vi "Measurement Logic.vi"() -> ()   [LabVIEW 2021, in "Noise Sweep_Class D Amplifier.lvlib"]
uses:
  Noise Sweep_Class D Amplifier.lvlib
  Measurement Configuration.ctl
  shared/DAQmx/input terminal configuration.ctl
  shared/controls/weighting filter.ctl
  Measurement Results.ctl
  <vilib>/MeasurementLink/MeasurementLink Measurement Server/Measure Call Context/Measure Call Context.lvclass
  <instrlib>/niDCPower/nidcpower.llb/niDCPower Source Mode.ctl
  <instrlib>/niDCPower/nidcpower.llb/niDCPower Output Function.ctl
  <instrlib>/niDCPower/nidcpower.llb/niDCPower Wait For Event - Event.ctl
  <vilib>/Analysis/1siggen.llb/Ramp Pattern by Samples.vi
  <vilib>/Analysis/5stat.llb/RMS (DBL).vi
  <vilib>/DAQmx/create/channels.llb/DAQmx Create Channel (AI-Voltage-Basic).vi
  <vilib>/DAQmx/configure/timing.llb/DAQmx Timing (Sample Clock).vi
  <vilib>/addons/Sound and Vibration/svt_Weighting/SVT A, B, C Weighting Filter (Fixed Rates) (N Ch).vi
  <vilib>/Analysis/NI_AALBase.lvlib
  <vilib>/addons/Sound and Vibration/svt_Weighting/SoundVib_ABCWeighting.lvlib
  <vilib>/Analysis/NI_AALPro.lvlib
  shared/DAQmx/DAQmx utility.lvlib
panel:
  out "XY Graph":cluster{"X data":dbl[], "Y data":dbl[]}[](graph)
  out "Waveform Graph":waveform(dbl)[](graph)
  out "measure call context out":refnum<class "Measure Call Context.lvclass">
  in  "measure call context in":refnum<class "Measure Call Context.lvclass">
  out "measurement results":T1={"channel names"=[], "power supply voltage (V)"=[], "idle channel noise (Vrms)"=[], "wfm - dt"=1.9531249997269942e-05, "wfm - data"=array[12800 elements]}
  in  "measurement configuration":T2={"acq channel"="PXI1Slot4/ai0", "acq sampling rate"=51200.0, "measurement time (s)"=0.1, "input range"=5.0, "input terminal cfg"=enum."Default", "weighting filter"=enum."A-weighting", "power supply resource"="PXI1Slot6", "power supply voltage start"=5.0, "power supply voltage stop"=14.0, "sweep number of steps"=10, "power supply current limit"=1.2}
  out "error out":errorcluster
  in  "error in":errorcluster
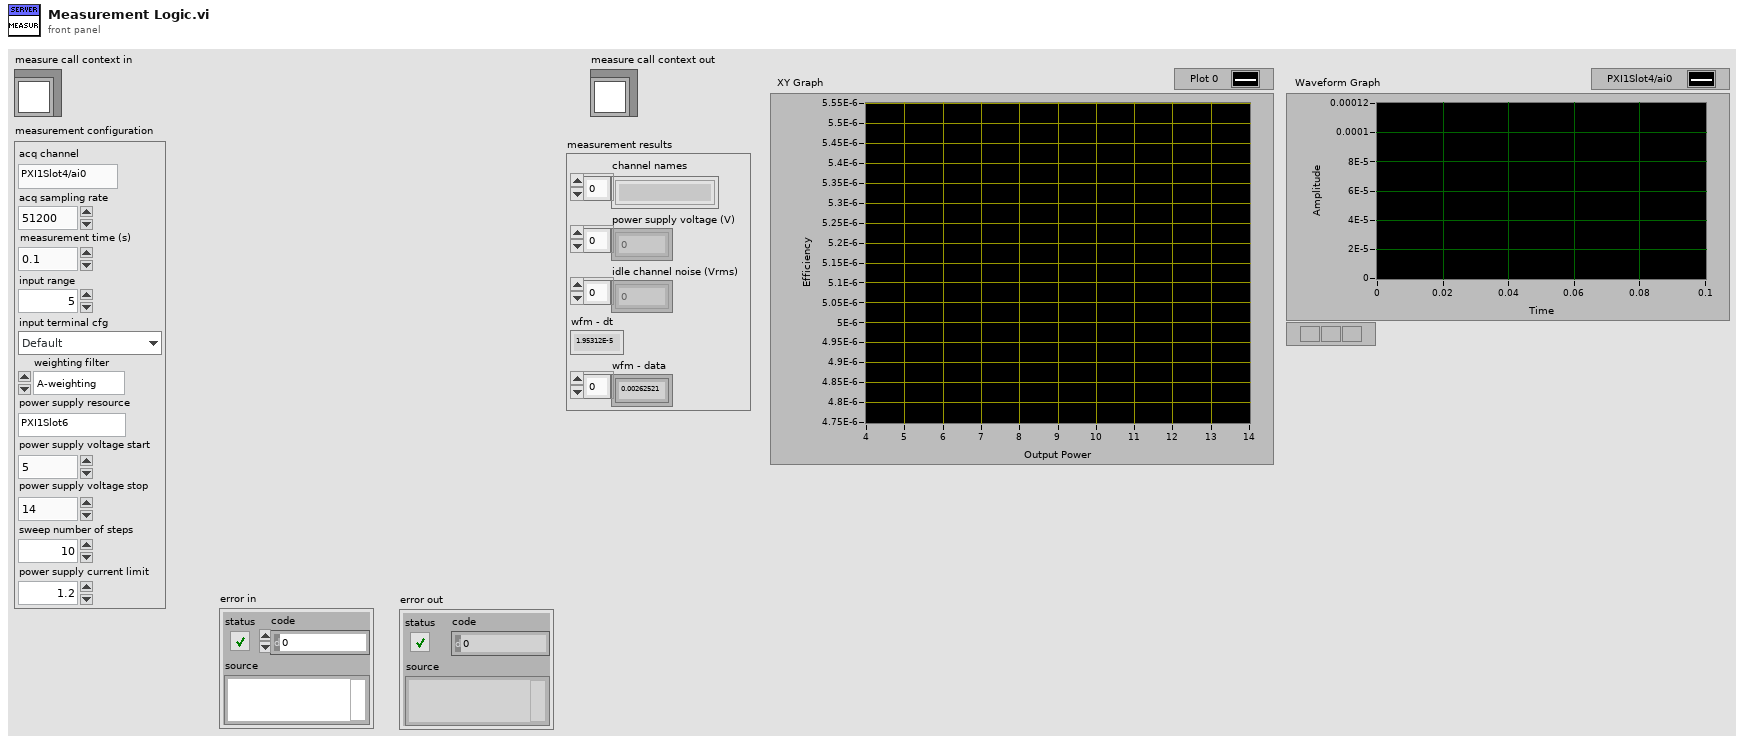
[diagram p1: front panel]
types:
  T1 = typedef "Noise Sweep_Class D Amplifier.lvlib/Measurement Results.ctl" = cluster{"channel names":string[], "power supply voltage (V)":dbl[], "idle channel noise (Vrms)":dbl[], "wfm - dt":dbl, "wfm - data":dbl[]}
  T2 = typedef "Noise Sweep_Class D Amplifier.lvlib/Measurement Configuration.ctl" = cluster{"acq channel":string, "acq sampling rate":dbl, "measurement time (s)":dbl, "input range":dbl, "input terminal cfg":T3, "weighting filter":T4, "power supply resource":string, "power supply voltage start":dbl, "power supply voltage stop":dbl, "sweep number of steps":u32, "power supply current limit":dbl}
  T3 = typedef "DAQmx utility.lvlib/input terminal configuration.ctl" = enum32{"Default", "NRSE", "RSE", "Differential", "Pseudodifferential"}
  T4 = typedef "weighting filter.ctl" = enum32{"Linear", "A-weighting", "B-weighting", "C-weighting"}
  T5 = typedef "niDCPower Output Function.ctl" = i32
  T6 = typedef "niDCPower Source Mode.ctl" = i32
  T7 = typedef "niDCPower Wait For Event - Event.ctl" = i32
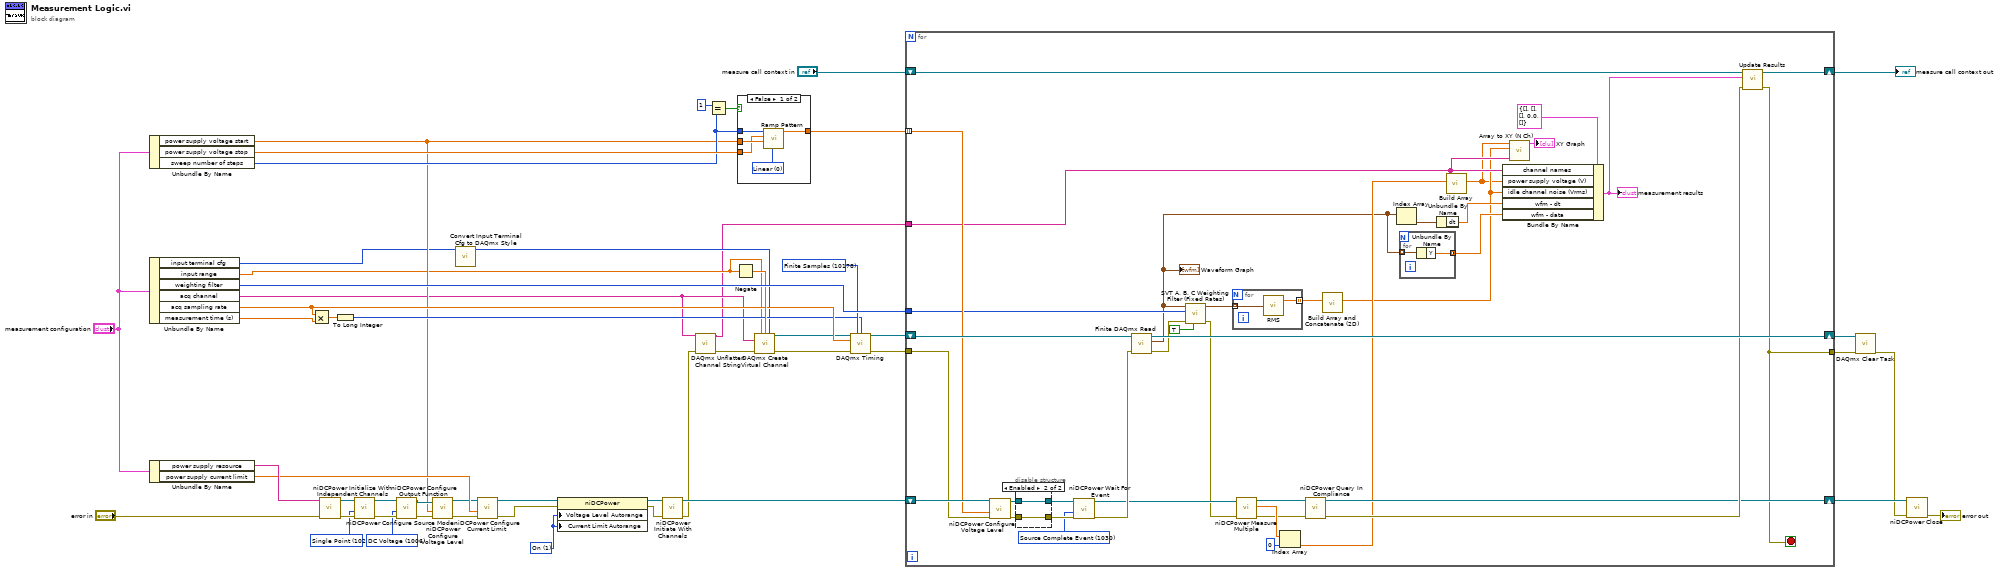
[diagram p0: block diagram]
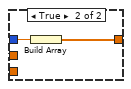
[diagram p2: hidden frame]
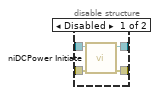
[diagram p3: hidden frame]
diagram:
  w18 = 10178 items=["Finite Samples"=10178, "Continuous Samples"=10123, "Hardware Timed Single Point"=12522] ("sample mode")
  w24 = 1 items=["Off", "On"] ("Source:DC Voltage:Current Limit Autorange")
  w25 = T5 1006 items=["DC Voltage"=1006, "DC Current"=1007, "Pulse Voltage"=1049, "Pulse Current"=1050] ("output function")
  w32 = T6 1020 items=["Single Point"=1020, "Sequence"=1021] ("source mode")
  n1 = Unbundle By Name("measurement configuration") -> ("power supply voltage start"=w12:dbl, "power supply voltage stop"=w23:dbl, "sweep number of steps"=w22:u32)
  n2 = Unbundle By Name("measurement configuration") -> ("input terminal cfg"=w9:T3, "input range"=w11:dbl, "weighting filter"=w21:T4, "acq channel"=w2:string, "acq sampling rate"=w16:dbl, "measurement time (s)"=w17:dbl)
  n3 = Unbundle By Name("measurement configuration") -> ("power supply resource"=w46:string, "power supply current limit"=w45:dbl)
  n4 = Multiply(x=w16, y=w17) -> (x*y=w15:dbl)
  n5 = call <instrlib>:"niDCPower Initialize With Independent Channels.vi"("error in (no error)"="error in", "resource name"=w46) -> ("error out"=w36:errorcluster, "instrument handle out"=w35:refnum<k15>)  [unwired: 8 in]
  n6 = To Long Integer(number=w15) -> (32bit integer=w14:i32)
  n7 = call <instrlib>:"niDCPower Configure Source Mode.vi"("error in (no error)"=w36, "source mode"=w32, "instrument handle"=w35) -> ("error out"=w34:errorcluster, "instrument handle out"=w33:refnum<k15>)  [unwired: 7 out]
  n8 = call <instrlib>:"niDCPower Configure Output Function.vi"("error in (no error)"=w34, "output function"=w25, "instrument handle"=w33) -> ("error out"=w26:errorcluster, "instrument handle out"=w27:refnum<k15>)  [unwired: 1 in, 6 out]
  n9 = call <instrlib>:"niDCPower Configure Voltage Level.vi"("error in (no error)"=w26, "voltage level"=w12, "instrument handle"=w27) -> ("error out"=w37:errorcluster, "instrument handle out"=w38:refnum<k15>)  [unwired: 1 in, 6 out]
  n10 = call "Convert Input Terminal Cfg to DAQmx Style.vi"("input terminal cfg"=w9) -> ("DAQmx input terminal cfg"=w10:i32)  [unwired: 10 in]
  n11 = call <instrlib>:"niDCPower Configure Current Limit.vi"("error in (no error)"=w37, "current limit"=w45, "instrument handle"=w38) -> ("error out"=w28:errorcluster, "instrument handle out"=w31:refnum<k15>)  [unwired: 2 in, 5 out]
  n12 = property class="niDCPower"(reference=w31, error in=w28, "Voltage Level Autorange"=w24, "Current Limit Autorange"=w24) -> (reference out=w30:refnum<k15>, error out=w29:errorcluster)
  n13 = call <instrlib>:"niDCPower Initiate With Channels.vi"("error in (no error)"=w29, "instrument handle"=w30) -> ("error out"=w4:errorcluster, "instrument handle out"=w41:refnum<k15>)  [unwired: 8 in]
  n14 = call <vilib>:"DAQmx Unflatten Channel String.vi"("names in"=w2, "error in"=w4) -> ("names out"=w1:string[], "error out"=w3:errorcluster)  [unwired: 12 in]
  n15 = Equal?(x=u32 1, y=w22) -> (x = y?=w49:bool)
  n16 = Negate(x=w11) -> (-x=w19:dbl)
  n17 = case shown="False" w49 {
    tunnel: w12 -> [w56 w58]
    tunnel: w23 -> [w55 _]
    tunnel: w22 -> [w54 _]
    tunnel: [w53 w57] -> w51
    frame False {
      w52 = u16 0 items=["Linear", "Logarithmic"] ("type")
      n18 = call-poly <vilib>:"Ramp Pattern.vi"("type"=w52, "start"=w56, "end"=w55, "samples"=w54) -> ("Ramp Pattern"=w53:dbl[])  [unwired: 6 in, 1 out]
    }
    frame True {
      n19 = Build Array(w58) -> (w57:dbl[])
    }
  }
  n20 = call-poly <vilib>:"DAQmx Create Virtual Channel.vi"("maximum value"=w11, "minimum value"=w19, "input terminal configuration"=w10, "physical channels"=w2, "error in"=w3) -> ("task out"=w8:refnum<k21>, "error out"=w7:errorcluster)  [unwired: 9 in]
  n21 = call-poly <vilib>:"DAQmx Timing.vi"("task/channels in"=w8, "sample mode"=w18, "samples per channel"=w14, "rate"=w16, "error in"=w7) -> ("task out"=w6:refnum<k21>, "error out"=w5:errorcluster)  [unwired: 9 in]
  n22 = for {
    tunnel: w51 -> [w86] mode=indexing
    shift-right: [w96] -> w50
    shift-left: "measure call context in" -> [w95]
    shift-right: [w75] -> w42
    shift-left: w41 -> [w88]
    shift-right: [w93] -> w40
    shift-left: w6 -> [w92]
    tunnel: w5 -> [w87]
    tunnel: w21 -> [w72]
    tunnel: [w71] -> w13
    tunnel: w1 -> [w62]
    stop <- w71 stop-if-true
    w83 = T7 1030 items=["Source Complete Event"=1030, "Measure Complete Event"=1031, "Sequence Iteration Complete Event"=1032, "Sequence Engine Done Event"=1033] ("event")
    n23 = call <instrlib>:"niDCPower Configure Voltage Level.vi"("error in (no error)"=w87, "voltage level"=w86, "instrument handle"=w88) -> ("error out"=w82:errorcluster, "instrument handle out"=w81:refnum<k15>)  [unwired: 1 in, 6 out]
    n24 = disable-structure shown="Enabled" {
      disable-tunnel: [w102 w104] -> w85
      disable-tunnel: [w101 w103] -> w84
      disable-tunnel: w82 -> [w100 w103]
      disable-tunnel: w81 -> [w99 w104]
      frame Disabled {
        n25 = call <instrlib>:"niDCPower Initiate.vi"("error in (no error)"=w100, "instrument handle"=w99) -> ("error out"=w101:errorcluster, "instrument handle out"=w102:refnum<k15>)  [unwired: 2 in, 6 out]
      }
      frame Enabled {
      }
    }
    n26 = call <instrlib>:"niDCPower Wait For Event.vi"("error in (no error)"=w84, "event"=w83, "instrument handle"=w85) -> ("error out"=w80:errorcluster, "instrument handle out"=w79:refnum<k15>)  [unwired: 1 in, 6 out]
    n27 = call "Finite DAQmx Read.vi"("error in (no error)"=w80, "task/channels in"=w92) -> ("error out"=w74:errorcluster, "data"=w65:waveform(dbl)[], "task out"=w93:refnum<k21>)  [unwired: 7 in]
    "Waveform Graph" <- w65
    n28 = call-poly <vilib>:"SVT A, B, C Weighting Filter (Fixed Rates).vi"("reset filter (F)"=TRUE, "error in (no error)"=w74, "weighting"=w72, "scaled signals [EU]"=w65) -> ("error out"=w73:errorcluster, "weighted signals [EU]"=w69:waveform(dbl)[])  [unwired: 5 in]
    n29 = for {
      tunnel: w69 -> [w106] mode=indexing
      tunnel: [w105] -> w63 mode=indexing
      n30 = call-poly <vilib>:"RMS.vi"("X"=w106) -> ("rms value"=w105:dbl)  [unwired: 1 out]
    }
    n31 = call <instrlib>:"niDCPower Measure Multiple.vi"("error in (no error)"=w73, "instrument handle"=w79) -> ("error out"=w78:errorcluster, "voltage measurements"=w89:dbl[], "instrument handle out"=w76:refnum<k15>)  [unwired: 6 in, 1 out]
    n32 = Index Array(array=w89, index=0) -> (element=w67:dbl)
    n33 = call <instrlib>:"niDCPower Query In Compliance.vi"("error in (no error)"=w78, "instrument handle"=w76) -> ("error out"=w77:errorcluster, "instrument handle out"=w75:refnum<k15>)  [unwired: 1 in, 7 out]
    n34 = call "Build Array and Concatenate (2D).vi"("Array"=w63) -> ("Array Out"=w60:dbl[])  [unwired: 10 in]
    n35 = Index Array(array=w65) -> (element=w68:waveform(dbl))  [unwired: 1 in]
    n36 = for {
      tunnel: w65 -> [w98] mode=indexing
      tunnel: [w97] -> w64 mode=concatenating
      n37 = Unbundle By Name(w98) -> ("Y"=w97:dbl[])
    }
    n38 = Unbundle By Name(w68) -> ("dt"=w66:dbl)
    n39 = call "Build Array.vi"("value"=w67) -> ("Array"=w59:dbl[])  [unwired: 10 in]
    n40 = Bundle By Name(cluster=T1 {"channel names"=[], "power supply voltage (V)"=[], "idle channel noise (Vrms)"=[], "wfm - dt"=0.0, "wfm - data"=[]} ("Measurement Results"), "channel names"=w62, "power supply voltage (V)"=w59, "idle channel noise (Vrms)"=w60, "wfm - dt"=w66, "wfm - data"=w64) -> (w94:T1)
    "measurement results" <- w94
    n41 = call "Array to XY (N Ch).vi"("channel names"=w62, "Y data"=w60, "X data"=w59) -> ("XY plots"=→"XY Graph":cluster{"X data":dbl[], "Y data":dbl[]}[])  [unwired: 8 in]
    n42 = call <vilib>:"Update Results.vi"("error in"=w77, "measurement results"=w94, "measure call context in"=w95) -> ("error out"=w71:errorcluster, "measure call context out"=w96:refnum<class "Measure Call Context.lvclass">)  [unwired: 7 in]
  }
  "measure call context out" <- w50
  n43 = call <vilib>:"DAQmx Clear Task.vi"("task in"=w40, "error in"=w13) -> ("error out"=w39:errorcluster)  [unwired: 13 in]
  n44 = call <instrlib>:"niDCPower Close.vi"("error in (no error)"=w39, "instrument handle"=w42) -> ("error out"=→"error out":errorcluster)  [unwired: 9 out]
